vi "get index of tag mapped to channel.vi"(9 "channel":refnum<class "TBM channel.lvclass">, 10 "owner":string, 11 "engine configuration in":refnum<class "engine configuration.lvclass">) -> (3 "tag index":i32)   [LabVIEW 2013, in "engine configuration.lvclass"]
uses:
  engine configuration.lvclass
  <vilib>/NI/Tag Bus Module Framework/channel/TBM channel.lvclass
  engine configuration.lvclass/engine configuration.ctl
  <vilib>/NI/Tag Bus Module Framework/channel/TBM channel.lvclass/TBM channel.ctl
  <vilib>/NI/Tag Bus/tag/tag descriptor.lvclass/tag descriptor.ctl
  <vilib>/NI/Tag Bus Module Framework/channel/Read channel classification.vi
  <vilib>/NI/Tag Bus/tag/read tag name.vi
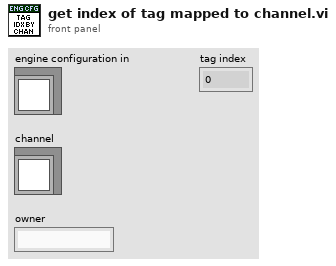
[diagram p1: front panel]
types:
  T1 = typedef "TBM channel.lvclass/channel classification.ctl" = enum16{"input data", "output data", "processing parameter", "processing result"}
  T2 = typedef "engine configuration.lvclass/module channel pairings.ctl" = cluster{"modules":string[], "channels":string[]}
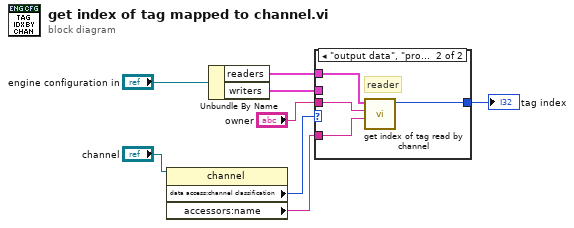
[diagram p0: block diagram]
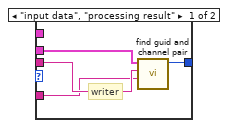
[diagram p2: hidden frame]
diagram:
  n1 = property class="channel"(reference="channel") -> ("data access:channel classification"=w4:T1, "accessors:name"=w7:string)  [unwired: 1 in, 2 out]
  n2 = Unbundle By Name("engine configuration in") -> ("readers"=w3:T2[], "writers"=w2:T2)
  n3 = case shown="\"output data\", \"processing parameter\"" w4 {
    tunnel: w2 -> [w11 _]
    tunnel: w3 -> [_ w14]
    tunnel: [w12 w15] -> w5
    tunnel: "owner" -> [w10 w13]
    tunnel: w7 -> [w9 w16]
    frame "input data", "processing result" {
      # "writer"
      n4 = call "find guid and channel pair.vi"("channel name"=w9, "Module GUID"=w10, "listing"=w11) -> ("index"=w12:i32)  [unwired: 8 in]
    }
    frame "output data", "processing parameter" {
      # "reader"
      n5 = call "get index of tag read by channel.vi"("channel"=w16, "module guid"=w13, "readers"=w14) -> ("tag index"=w15:i32)  [unwired: 8 in]
    }
  }
  "tag index" <- w5
